vi "SENS_CORR_COLL_SESS_DESC.vi"(0 "VISA IN":refnum<visa-resource-name>, 5 "error in":errorcluster, 7 "Channel":i32, 9 "Session":i32, 11 "StepNum":i32) -> (14 "VISA Out":refnum<visa-resource-name>, 16 "read buffer":string, 19 "error out":errorcluster)   [LabVIEW 2018, in "PNA-X.lvlib"]
doc: "SENS:CORR:COLL:SESS6:DESC?"
uses:
  PNA-X.lvlib
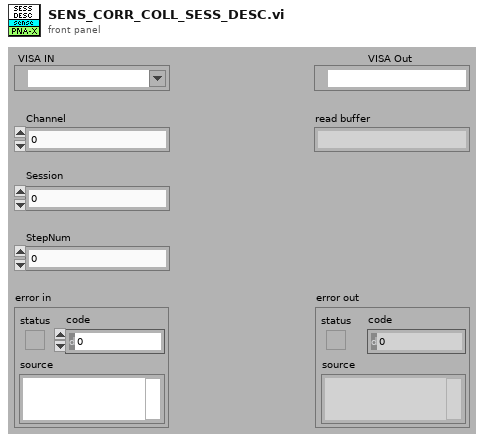
[diagram p1: front panel]
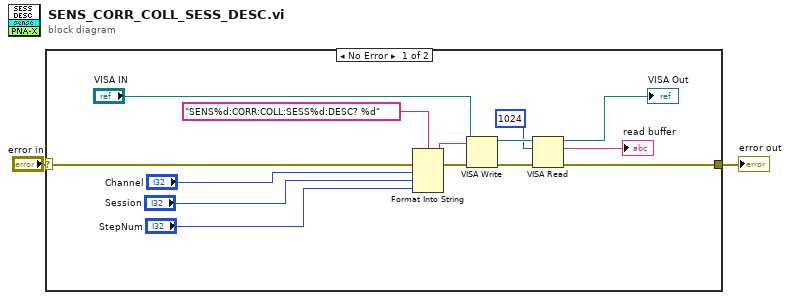
[diagram p0: block diagram]
diagram:
  n1 = case shown="No Error" "error in" {
    selector: "error in" -> [w16 w17]
    tunnel: [w4 w17] -> w1
    frame No Error {
      n2 = Format Into String(format string="SENS%d:CORR:COLL:SESS%d:DESC? %d" ("Cmdline"), error in=w16, "Channel", "Session", "StepNum") -> (resulting string=w14:string, error out=w15:errorcluster)  [unwired: 1 in]
      n3 = VISA Write(VISA resource name="VISA IN", write buffer=w14, error in (no error)=w15) -> (VISA resource name out=w8:refnum<visa-resource-name>, error out=w7:errorcluster)  [unwired: 1 out]
      n4 = VISA Read(VISA resource name=w8, byte count=u32 1024, error in (no error)=w7) -> (VISA resource name out=→"VISA Out":refnum<visa-resource-name>, read buffer=→"read buffer":string, error out=w4:errorcluster)  [unwired: 1 out]
    }
    frame Error {
    }
  }
  "error out" <- w1
